vi "FTW-Subscriber-Construct.vi"(5 "Publisher Address":string, 7 "Receive Message Size Limit":i32=1000 format="%_4pbytes", 9 "Linger":i32=200 format="%d msec", 11 "error in":errorcluster) -> (4 "FTW Subscriber":refnum<data-value>, 6 "Subscription":refnum<event-registration>, 15 "error out":errorcluster)   [LabVIEW 2014]
uses:
  core/FTW-Subscriber-Core-Type.ctl
  error/FTW-ERR-ThrowGenericError.vi
  error/FTW-ERR-ThrowError.vi
  error/FTW-ERR-NoErrorConstant.vi
  error/FTW-ERR-CallChain.vi
  string/FTW-STR-ReplaceWhitespace.vi
panel:
  # "Inputs"
  # "Outputs"
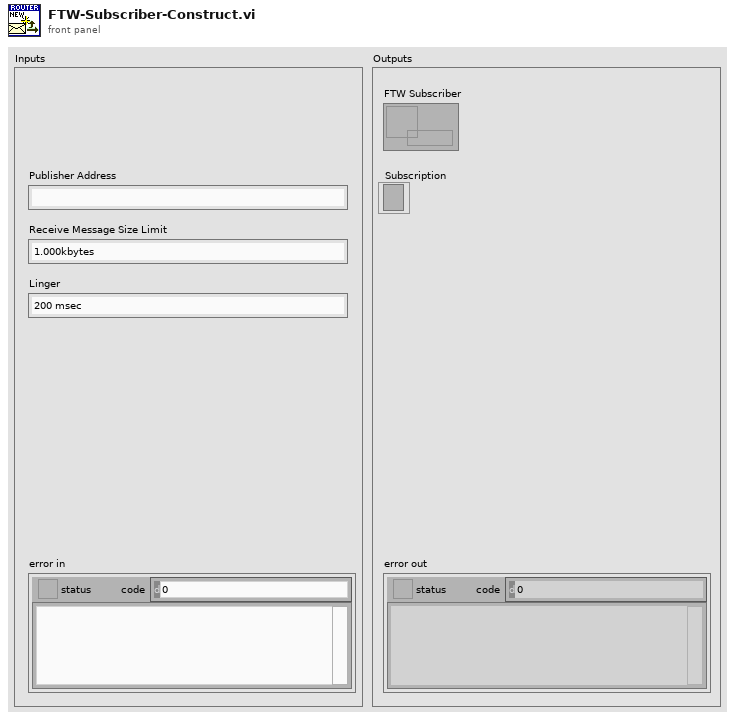
[diagram p1: front panel]
types:
  T1 = typedef "FTW-Subscriber-Core-Type.ctl" = cluster{"Socket":i64, "SubscriptionEvent":refnum<user-event>}
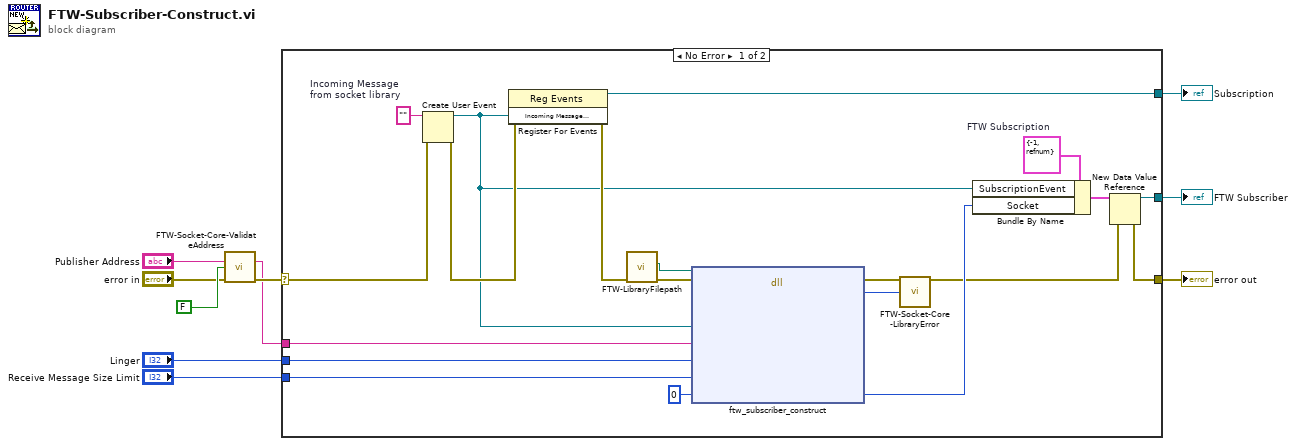
[diagram p0: block diagram]
diagram:
  n1 = call "FTW-Socket-Core-ValidateAddress.vi"("Address"="Publisher Address", "Allow wildcard replacement?"=FALSE, "error in"="error in") -> ("Sanitized Address"=w6:string, "error out"=w8:errorcluster)  [unwired: 10 in, 1 out]
  n2 = case shown="No Error" w8 {
    selector: w8 -> [w16 w31]
    tunnel: [w22 _] -> w10
    tunnel: [w20 w31] -> w9
    tunnel: [w13 _] -> w4
    tunnel: w6 -> [w27 _]
    tunnel: "Linger" -> [w19 _]
    tunnel: "Receive Message Size Limit" -> [w18 _]
    frame No Error {
      w12 = T1 {"Socket"=-1, "SubscriptionEvent"=refnum}  # FTW Subscription
      w17 = ""  # Incoming Message from socket library
      n3 = Create User Event(user event datatype=w17, error in=w16) -> (user event=w11:refnum<user-event>, error out=w15:errorcluster)
      n4 = register-events(error in=w15, w11) -> (reference out=w13:refnum<event-registration>, error out=w14:errorcluster)  [unwired: 1 in]
      n5 = call "FTW-LibraryFilepath.vi"("error in"=w14) -> ("error out"=w29:errorcluster, "Library Filepath"=w30:path)  [unwired: 8 in, 1 out]
      n6 = dll-call lib="?" fn="ftw_subscriber_construct"(path in=w30, error in=w29, "Incoming Message Event"=w11, "Address"=w27, "Linger (msec)"=w19, "Max Recv Size (bytes)"=w18, "Socket Handle"=i64 0) -> (error out=w28:errorcluster, "Return Value"=w26:i64, "Socket Handle"=w24:i64)  [unwired: 7 in, 1 out]
      n7 = call "FTW-Socket-Core-LibraryError.vi"("error in"=w28, "Return Value"=w26) -> ("error out"=w21:errorcluster)  [unwired: 13 in]
      n8 = Bundle By Name(cluster=w12, "SubscriptionEvent"=w11, "Socket"=w24) -> (w23:T1)
      n9 = New Data Value Reference(data value=w23, error in=w21) -> (data value reference=w22:refnum<data-value>, error out=w20:errorcluster)
    }
    frame Error {
    }
  }
  "error out" <- w9
  "FTW Subscriber" <- w10
  "Subscription" <- w4
